vi "Read uid.vi"(8 "error in (no error)":errorcluster, 11 "PersistentObject in":refnum<class "PersistentObject.lvclass">) -> (0 "error out":errorcluster, 2 "uid":u64, 3 "PersistentObject out":refnum<class "PersistentObject.lvclass">)   [LabVIEW 2018, in "PersistentObject.lvclass"]
uses:
  PersistentObject.lvclass
  PersistentObject.lvclass/PersistentObject.ctl
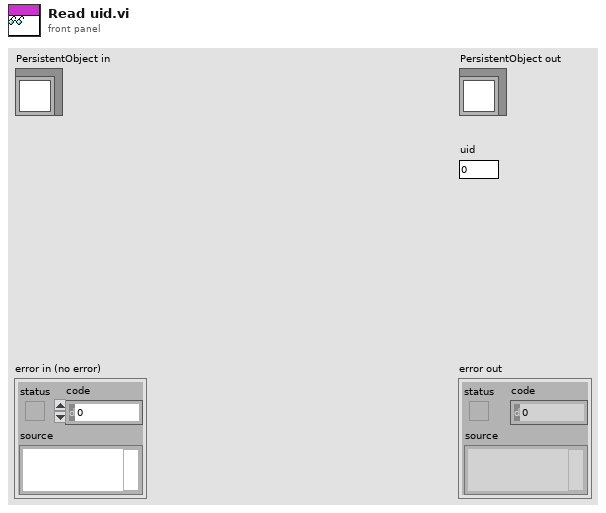
[diagram p1: front panel]
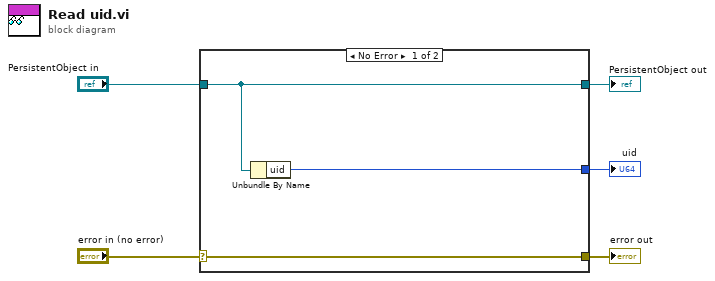
[diagram p0: block diagram]
diagram:
  n1 = case shown="No Error" "error in (no error)" {
    selector: "error in (no error)" -> [w8 w9]
    tunnel: [w8 w9] -> w4
    tunnel: [w7 w10] -> w2
    tunnel: "PersistentObject in" -> [w7 w10]
    tunnel: [w6 _] -> w1
    frame No Error {
      n2 = Unbundle By Name(w7) -> ("uid"=w6:u64)
    }
    frame Error {
    }
  }
  "error out" <- w4
  "PersistentObject out" <- w2
  "uid" <- w1
